vi "atm1.vi"() -> ()   [LabVIEW 2021]
uses:
  Control 8.ctl
  <vilib>/Utility/miscctls.llb/LVPointTypeDef.ctl
panel:
  in  "停止":bool
  in  "插入卡片":bool caption="Card"
  in  "密碼":string
  in  "error in (no error)":errorcluster
  out "error out":errorcluster
  in  "取消":bool
  in  "登入":bool
  in  "帳戶":bool
  in  "領取":bool
  in  "存入":bool
  in  "Money":i32
  out "提示和信息":string
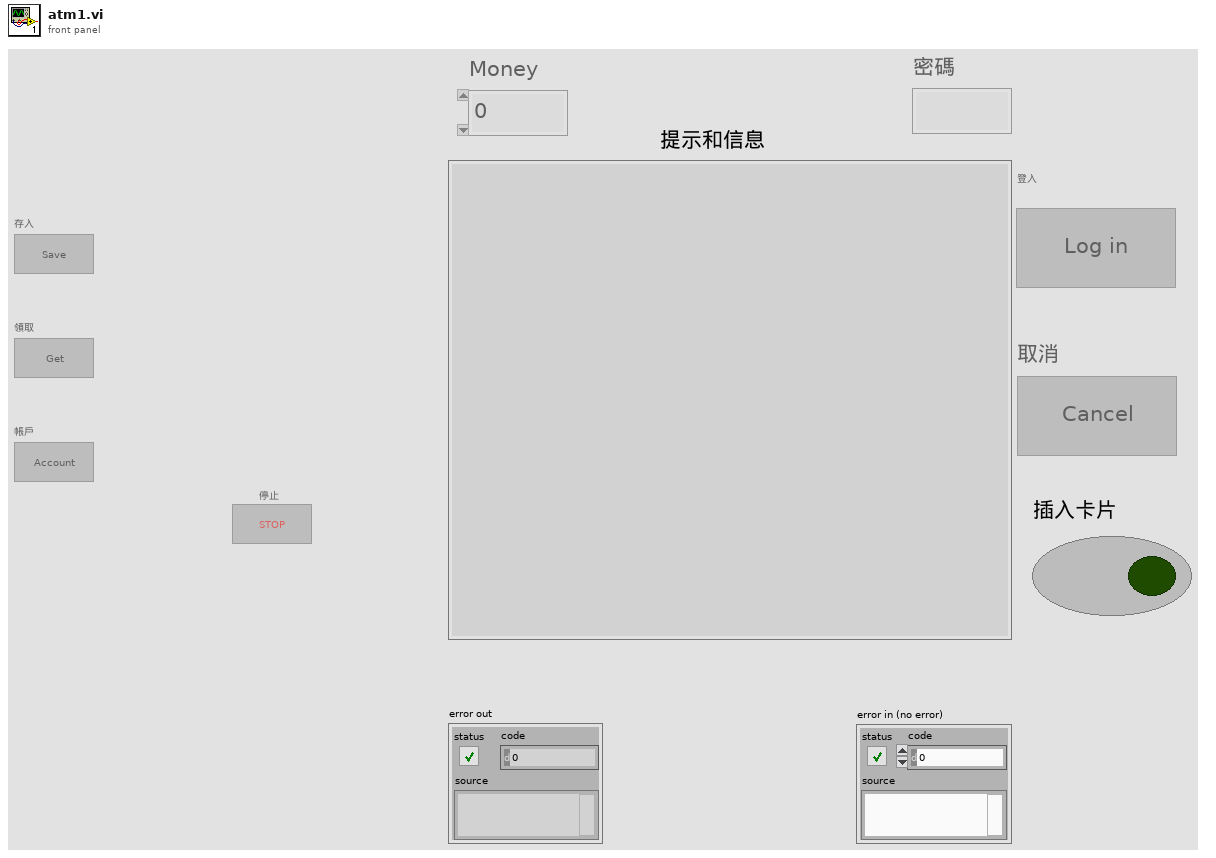
[diagram p1: front panel]
types:
  T1 = typedef "Control 8.ctl" = enum16{"初始化", "調整按鈕狀態", "等待事件", "插入卡片", "登入成功", "密碼錯誤", "密碼連續錯誤", "提款檢查", "提款成功", "提款失敗", "存款", "查詢帳戶餘額", "取消交易", "更新訊息", "停止程式"}
  T2 = typedef "LVPointTypeDef.ctl" = cluster{"Horizontal":i16, "Vertical":i16}
  T3 = enum16{"Enabled", "Disabled", "Disabled and Grayed Out"}
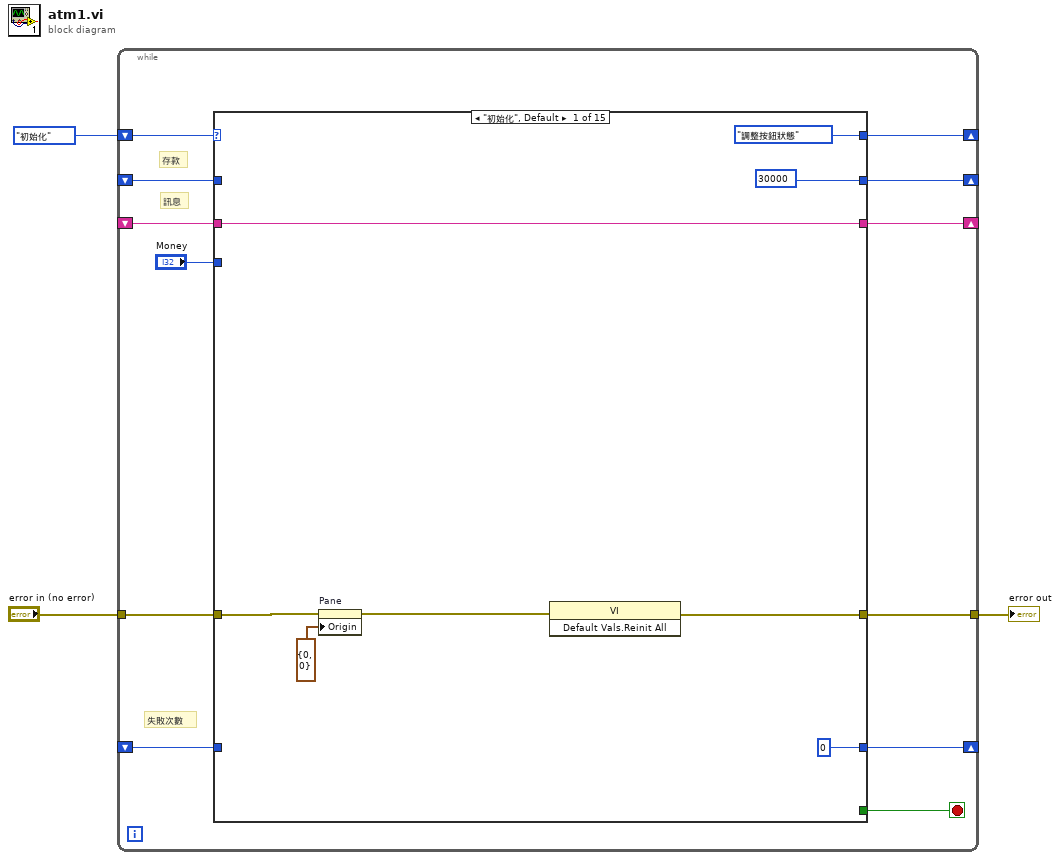
[diagram p0: block diagram]
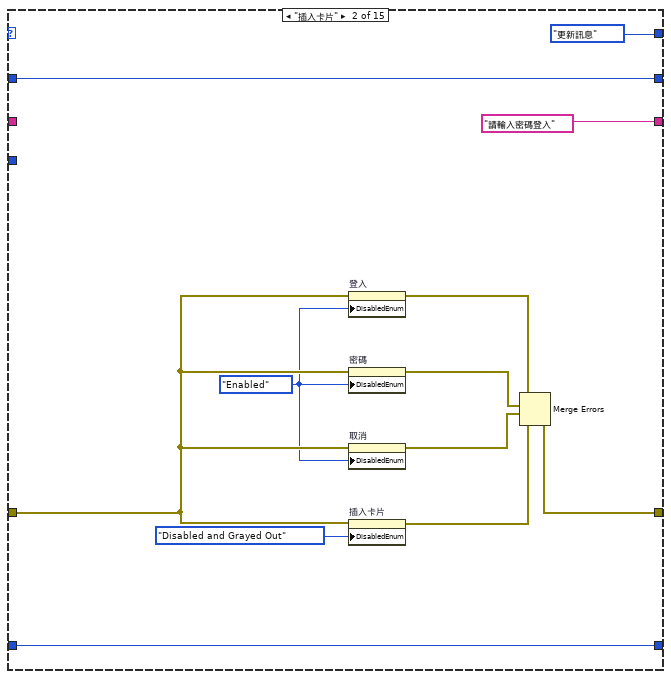
[diagram p2: hidden frame]
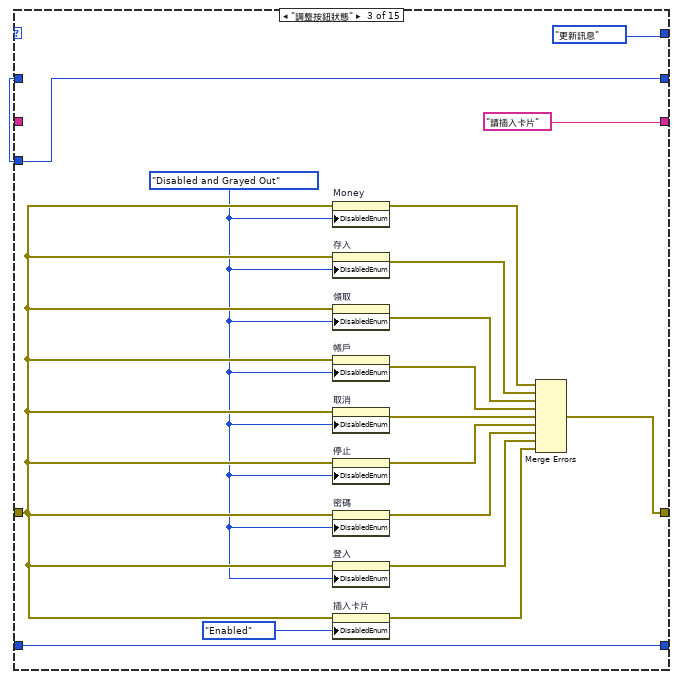
[diagram p3: hidden frame]
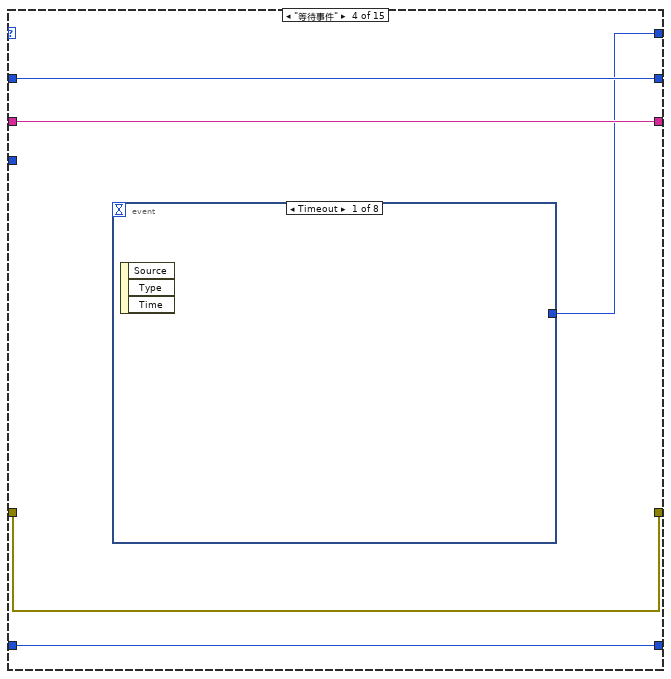
[diagram p4: hidden frame]
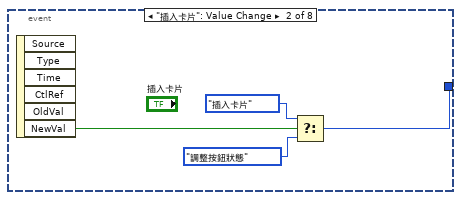
[diagram p5: hidden frame]
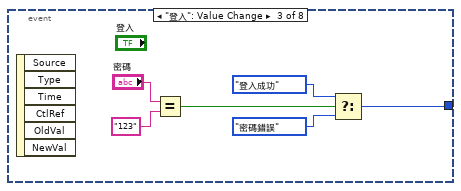
[diagram p6: hidden frame]
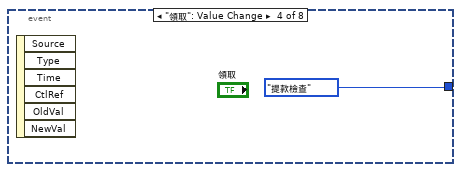
[diagram p7: hidden frame]
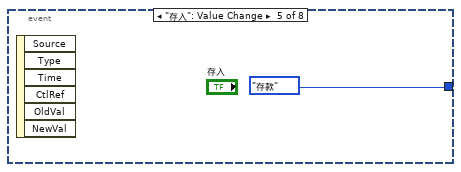
[diagram p8: hidden frame]
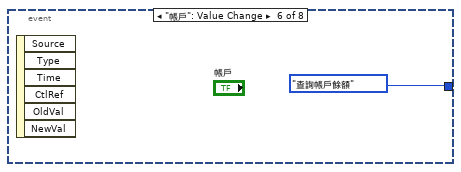
[diagram p9: hidden frame]
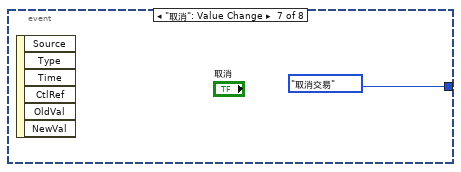
[diagram p10: hidden frame]
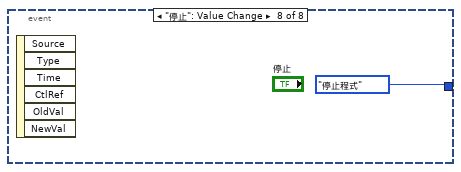
[diagram p11: hidden frame]
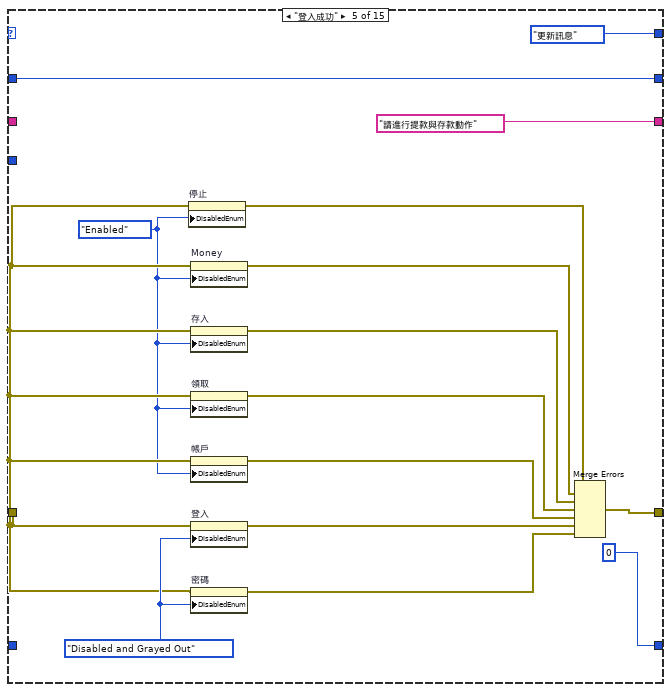
[diagram p12: hidden frame]
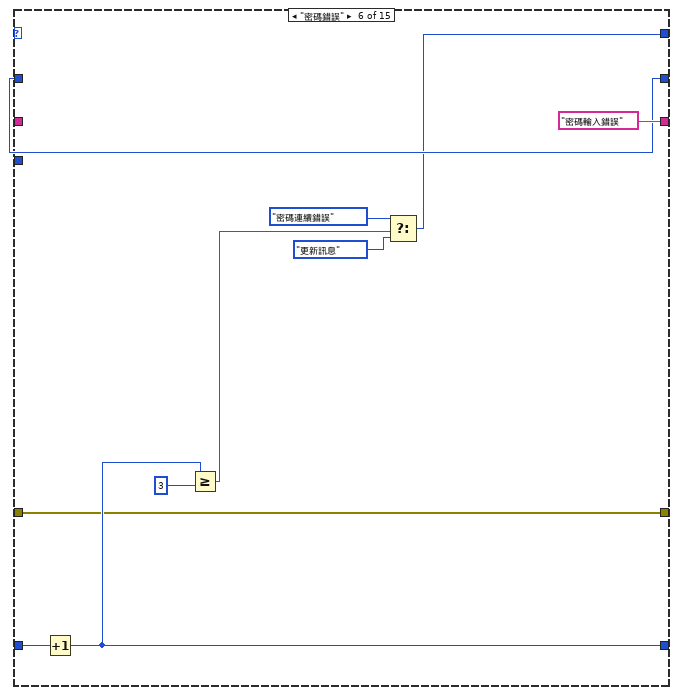
[diagram p13: hidden frame]
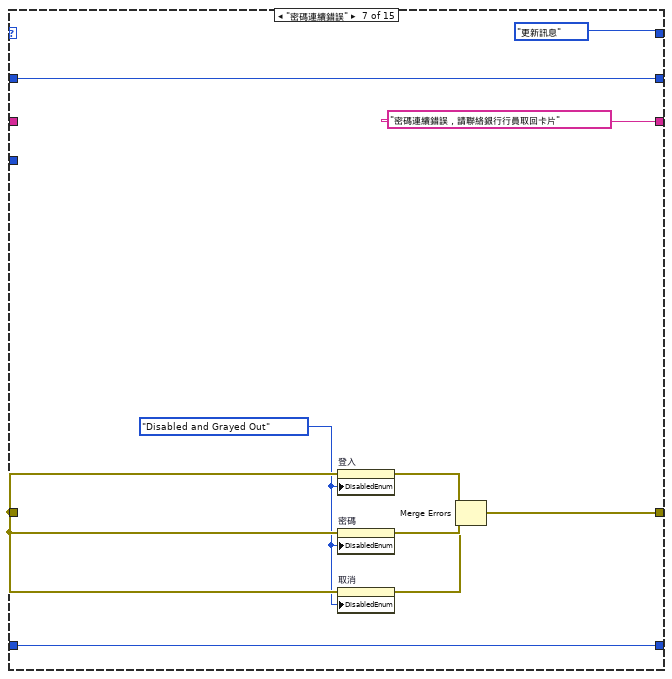
[diagram p14: hidden frame]
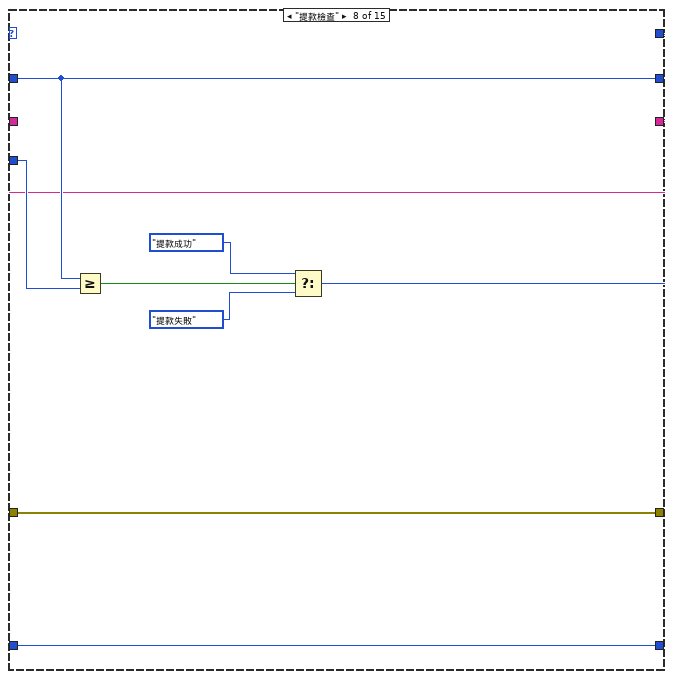
[diagram p15: hidden frame]
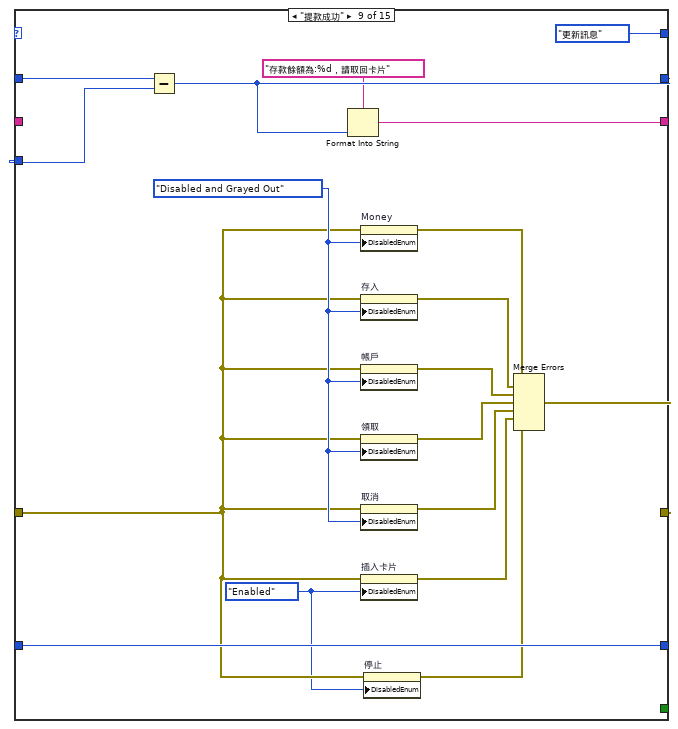
[diagram p16: hidden frame]
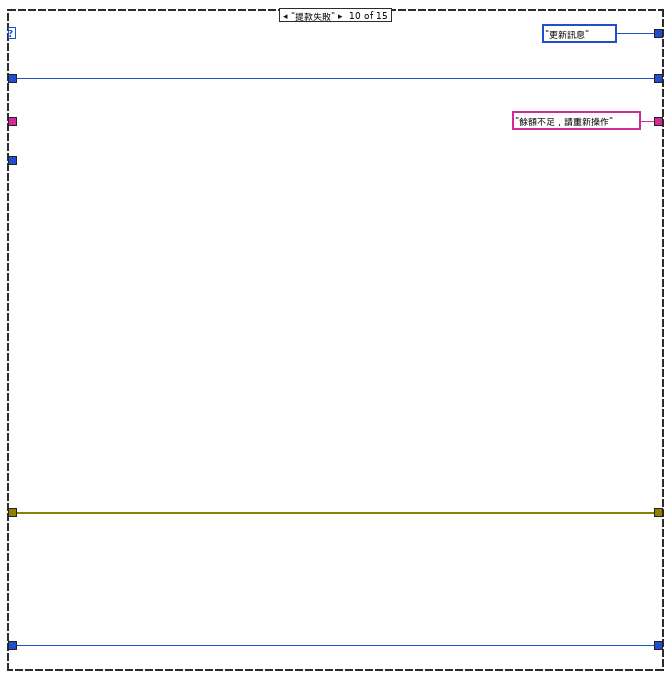
[diagram p17: hidden frame]
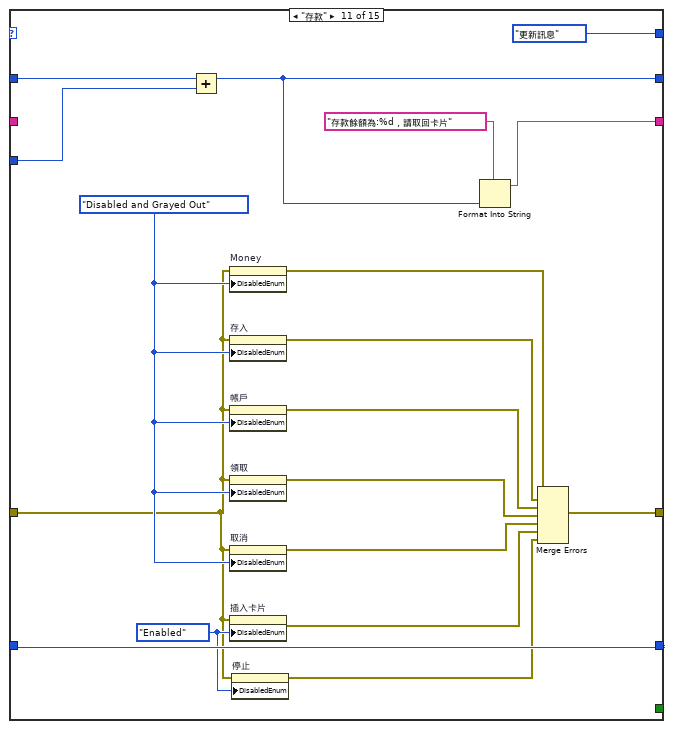
[diagram p18: hidden frame]
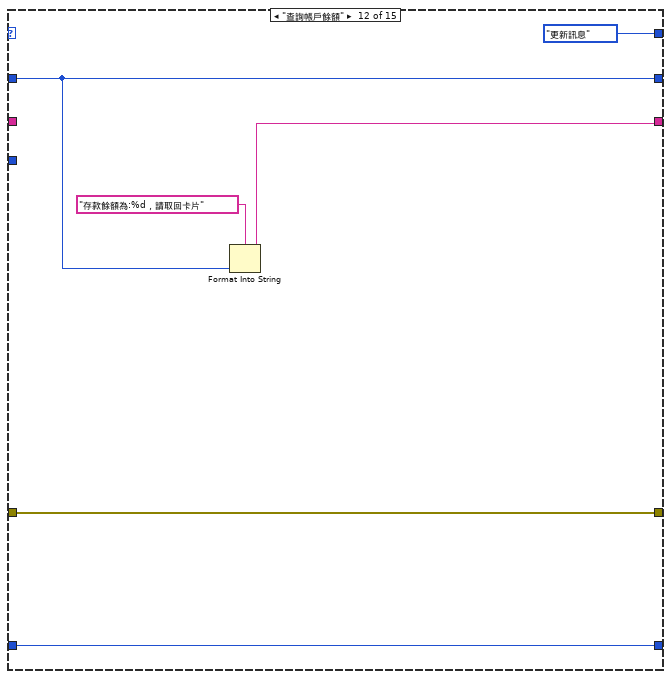
[diagram p19: hidden frame]
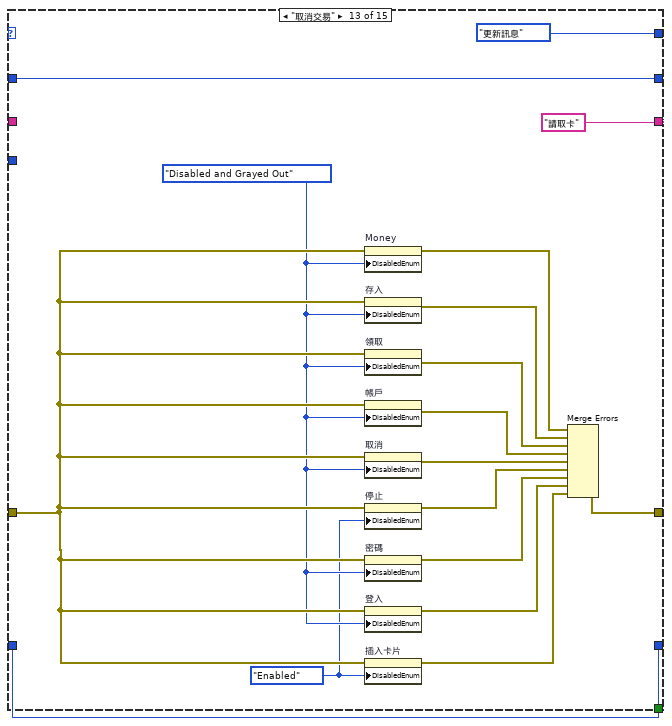
[diagram p20: hidden frame]
diagram:
  n1 = while {
    tunnel: "error in (no error)" -> [w9]
    shift-right: [w12] -> _
    shift-left: _ -> [w15]
    shift-right: [w8] -> _
    shift-left: _ -> [w14]
    shift-right: [w13] -> _
    shift-left: _ -> [w7]
    tunnel: [w10] -> w2
    shift-right: [w5] -> _
    shift-left: Control_8."初始化" -> [w6]
    stop <- w4 stop-if-true
    # "存款"
    # "訊息"
    # "失敗次數"
    n2 = case shown="\"初始化\", Default" w6 {
      selector: w6 -> [_ _ _ _ _ _ _ _ _ _ _ _ _ _ w194]
      tunnel: w15 -> [_ w30 w38 w55 w87 w92 w107 w113 w127 w138 w156 w160 w168 w187 w193]
      tunnel: w14 -> [w17 _ _ w54 _ _ _ w110 _ _ _ _ _ w185 w192]
      tunnel: [0 w27 w40 w57 0 w94 w99 w108 w129 w135 w144 w158 w169 w183 w189] -> w13
      tunnel: [30000 w30 w38 w55 w87 w92 w107 w113 w125 w138 w152 w160 w168 w187 w193] -> w12
      tunnel: "Money" -> [_ _ _ _ _ _ _ w114 w126 _ w155 _ _ _ _]
      tunnel: [w22 w26 w41 w56 w77 w90 w102 w109 w128 w136 w145 w159 w170 w184 w190] -> w10
      tunnel: w9 -> [w21 w35 w51 w56 w74 w90 w106 w109 w120 w136 w141 w159 w171 w184 w191]
      tunnel: [w17 "請輸入密碼登入" "請插入卡片" w54 "請進行提款與存款動作" "密碼輸入錯誤" "密碼連續錯誤，請聯絡銀行行員取回卡片" w110 w123 "餘額不足，請重新操作" w154 w161 "請取卡" w185 w192] -> w8
      tunnel: w7 -> [_ w27 w40 w57 _ w95 w99 w108 w129 w135 w144 w158 w169 w183 w189]
      tunnel: [Control_8."調整按鈕狀態" Control_8."更新訊息" Control_8."更新訊息" w53 Control_8."更新訊息" w91 Control_8."更新訊息" w111 Control_8."更新訊息" Control_8."更新訊息" Control_8."更新訊息" Control_8."更新訊息" Control_8."更新訊息" Control_8."等待事件" w194] -> w5
      tunnel: [_ _ _ _ _ _ _ _ _ _ _ _ _ _ TRUE] -> w4
      frame "初始化", Default {
        n3 = property on="Pane" class="Pane"(error in=w21, "Origin"=T2 {"Horizontal"=0, "Vertical"=0}) -> (error out=w20:errorcluster)  [unwired: 1 in, 1 out]
        n4 = invoke class="VI" method="Default Vals.Reinit All"(error in=w20) -> (error out=w22:errorcluster)  [unwired: 2 in, 2 out]
      }
      frame "插入卡片" {
        w25 = T3."Enabled"
        n5 = property on="登入" class="Bool"(error in=w35, "DisabledEnum"=w25) -> (error out=w34:errorcluster)  [unwired: 1 in, 1 out]
        n6 = property on="密碼" class="Str"(error in=w35, "DisabledEnum"=w25) -> (error out=w33:errorcluster)  [unwired: 1 in, 1 out]
        n7 = property on="取消" class="Bool"(error in=w35, "DisabledEnum"=w25) -> (error out=w32:errorcluster)  [unwired: 1 in, 1 out]
        n8 = property on="插入卡片" class="Bool (strict)"(error in=w35, "DisabledEnum"=T3."Disabled and Grayed Out") -> (error out=w31:errorcluster)  [unwired: 1 in, 1 out]
        n9 = Merge Errors(w34, w33, w32, w31) -> (w26:errorcluster)
      }
      frame "調整按鈕狀態" {
        w36 = T3."Disabled and Grayed Out"
        n10 = property on="Money" class="DigNum (strict)"(error in=w51, "DisabledEnum"=w36) -> (error out=w50:errorcluster)  [unwired: 1 in, 1 out]
        n11 = property on="存入" class="Bool"(error in=w51, "DisabledEnum"=w36) -> (error out=w49:errorcluster)  [unwired: 1 in, 1 out]
        n12 = property on="領取" class="Bool"(error in=w51, "DisabledEnum"=w36) -> (error out=w48:errorcluster)  [unwired: 1 in, 1 out]
        n13 = property on="帳戶" class="Bool"(error in=w51, "DisabledEnum"=w36) -> (error out=w47:errorcluster)  [unwired: 1 in, 1 out]
        n14 = property on="取消" class="Bool"(error in=w51, "DisabledEnum"=w36) -> (error out=w46:errorcluster)  [unwired: 1 in, 1 out]
        n15 = property on="停止" class="Bool"(error in=w51, "DisabledEnum"=w36) -> (error out=w45:errorcluster)  [unwired: 1 in, 1 out]
        n16 = property on="密碼" class="Str"(error in=w51, "DisabledEnum"=w36) -> (error out=w44:errorcluster)  [unwired: 1 in, 1 out]
        n17 = property on="登入" class="Bool"(error in=w51, "DisabledEnum"=w36) -> (error out=w43:errorcluster)  [unwired: 1 in, 1 out]
        n18 = property on="插入卡片" class="Bool (strict)"(error in=w51, "DisabledEnum"=T3."Enabled") -> (error out=w42:errorcluster)  [unwired: 1 in, 1 out]
        n19 = Merge Errors(w50, w49, w48, w47, w46, w45, w44, w43, w42) -> (w41:errorcluster)
      }
      frame "等待事件" {
        n20 = event shown="[0] Timeout" {
          selector: _ -> [_ _ _ _ _ _ _ _]
          dyn-events: _ -> [_ _ _ _ _ _ _ _]
          timeout: _ -> [_ _ _ _ _ _ _ _]
          tunnel: [_ w58 w62 Control_8."提款檢查" Control_8."存款" Control_8."查詢帳戶餘額" Control_8."取消交易" Control_8."停止程式"] -> w53
          event Timeout {
            n21 = event-data() -> ()  [unwired: 1 in, 3 out]
          }
          event "插入卡片": Value Change {
            n22 = event-data() -> ("NewVal"=w59:bool)  [unwired: 1 in, 5 out]
            n23 = Select(t=Control_8."插入卡片", s=w59, f=Control_8."調整按鈕狀態") -> (s? t:f=w58:T1)
          }
          event "登入": Value Change {
            n24 = event-data() -> ()  [unwired: 1 in, 6 out]
            n25 = Equal?(x="密碼", y="123") -> (x = y?=w63:bool)
            n26 = Select(t=Control_8."登入成功", s=w63, f=Control_8."密碼錯誤") -> (s? t:f=w62:T1)
          }
          event "領取": Value Change {
            n27 = event-data() -> ()  [unwired: 1 in, 6 out]
          }
          event "存入": Value Change {
            n28 = event-data() -> ()  [unwired: 1 in, 6 out]
          }
          event "帳戶": Value Change {
            n29 = event-data() -> ()  [unwired: 1 in, 6 out]
          }
          event "取消": Value Change {
            n30 = event-data() -> ()  [unwired: 1 in, 6 out]
          }
          event "停止": Value Change {
            n31 = event-data() -> ()  [unwired: 1 in, 6 out]
          }
        }
      }
      frame "登入成功" {
        w76 = T3."Disabled and Grayed Out"
        w73 = T3."Enabled"
        n32 = property on="停止" class="Bool"(error in=w74, "DisabledEnum"=w73) -> (error out=w75:errorcluster)  [unwired: 1 in, 1 out]
        n33 = property on="Money" class="DigNum (strict)"(error in=w74, "DisabledEnum"=w73) -> (error out=w84:errorcluster)  [unwired: 1 in, 1 out]
        n34 = property on="存入" class="Bool"(error in=w74, "DisabledEnum"=w73) -> (error out=w83:errorcluster)  [unwired: 1 in, 1 out]
        n35 = property on="領取" class="Bool"(error in=w74, "DisabledEnum"=w73) -> (error out=w82:errorcluster)  [unwired: 1 in, 1 out]
        n36 = property on="帳戶" class="Bool"(error in=w74, "DisabledEnum"=w73) -> (error out=w81:errorcluster)  [unwired: 1 in, 1 out]
        n37 = property on="登入" class="Bool"(error in=w74, "DisabledEnum"=w76) -> (error out=w80:errorcluster)  [unwired: 1 in, 1 out]
        n38 = property on="密碼" class="Str"(error in=w74, "DisabledEnum"=w76) -> (error out=w79:errorcluster)  [unwired: 1 in, 1 out]
        n39 = Merge Errors(w75, w84, w83, w82, w81, w80, w79) -> (w77:errorcluster)
      }
      frame "密碼錯誤" {
        n40 = Increment(x=w95) -> (x+1=w94:i32)
        n41 = Greater Or Equal?(x=w94, y=3) -> (x >= y?=w93:bool)
        n42 = Select(t=Control_8."密碼連續錯誤", s=w93, f=Control_8."更新訊息") -> (s? t:f=w91:T1)
      }
      frame "密碼連續錯誤" {
        w98 = T3."Disabled and Grayed Out"
        n43 = property on="登入" class="Bool"(error in=w106, "DisabledEnum"=w98) -> (error out=w105:errorcluster)  [unwired: 1 in, 1 out]
        n44 = property on="密碼" class="Str"(error in=w106, "DisabledEnum"=w98) -> (error out=w104:errorcluster)  [unwired: 1 in, 1 out]
        n45 = property on="取消" class="Bool"(error in=w106, "DisabledEnum"=w98) -> (error out=w103:errorcluster)  [unwired: 1 in, 1 out]
        n46 = Merge Errors(w105, w104, w103) -> (w102:errorcluster)
      }
      frame "提款檢查" {
        n47 = Greater Or Equal?(x=w113, y=w114) -> (x >= y?=w112:bool)
        n48 = Select(t=Control_8."提款成功", s=w112, f=Control_8."提款失敗") -> (s? t:f=w111:T1)
      }
      frame "提款成功" {
        w121 = T3."Disabled and Grayed Out"
        w119 = T3."Enabled"
        n49 = Subtract(x=w127, y=w126) -> (x-y=w125:i32)
        n50 = Format Into String(format string="存款餘額為:%d，請取回卡片", w125) -> (resulting string=w123:string)  [unwired: 2 in, 1 out]
        n51 = property on="Money" class="DigNum (strict)"(error in=w120, "DisabledEnum"=w121) -> (error out=w134:errorcluster)  [unwired: 1 in, 1 out]
        n52 = property on="存入" class="Bool"(error in=w120, "DisabledEnum"=w121) -> (error out=w133:errorcluster)  [unwired: 1 in, 1 out]
        n53 = property on="帳戶" class="Bool"(error in=w120, "DisabledEnum"=w121) -> (error out=w132:errorcluster)  [unwired: 1 in, 1 out]
        n54 = property on="領取" class="Bool"(error in=w120, "DisabledEnum"=w121) -> (error out=w131:errorcluster)  [unwired: 1 in, 1 out]
        n55 = property on="取消" class="Bool"(error in=w120, "DisabledEnum"=w121) -> (error out=w130:errorcluster)  [unwired: 1 in, 1 out]
        n56 = property on="插入卡片" class="Bool (strict)"(error in=w120, "DisabledEnum"=w119) -> (error out=w118:errorcluster)  [unwired: 1 in, 1 out]
        n57 = property on="停止" class="Bool"(error in=w120, "DisabledEnum"=w119) -> (error out=w117:errorcluster)  [unwired: 1 in, 1 out]
        n58 = Merge Errors(w134, w133, w132, w131, w130, w118, w117) -> (w128:errorcluster)
      }
      frame "提款失敗" {
      }
      frame "存款" {
        w142 = T3."Enabled"
        w143 = T3."Disabled and Grayed Out"
        n59 = Add(x=w156, y=w155) -> (x+y=w152:i32)
        n60 = property on="Money" class="DigNum (strict)"(error in=w141, "DisabledEnum"=w143) -> (error out=w151:errorcluster)  [unwired: 1 in, 1 out]
        n61 = property on="存入" class="Bool"(error in=w141, "DisabledEnum"=w143) -> (error out=w150:errorcluster)  [unwired: 1 in, 1 out]
        n62 = property on="帳戶" class="Bool"(error in=w141, "DisabledEnum"=w143) -> (error out=w149:errorcluster)  [unwired: 1 in, 1 out]
        n63 = property on="領取" class="Bool"(error in=w141, "DisabledEnum"=w143) -> (error out=w148:errorcluster)  [unwired: 1 in, 1 out]
        n64 = property on="取消" class="Bool"(error in=w141, "DisabledEnum"=w143) -> (error out=w147:errorcluster)  [unwired: 1 in, 1 out]
        n65 = property on="插入卡片" class="Bool (strict)"(error in=w141, "DisabledEnum"=w142) -> (error out=w146:errorcluster)  [unwired: 1 in, 1 out]
        n66 = property on="停止" class="Bool"(error in=w141, "DisabledEnum"=w142) -> (error out=w140:errorcluster)  [unwired: 1 in, 1 out]
        n67 = Format Into String(format string="存款餘額為:%d，請取回卡片", w152) -> (resulting string=w154:string)  [unwired: 2 in, 1 out]
        n68 = Merge Errors(w151, w150, w149, w148, w147, w146, w140) -> (w145:errorcluster)
      }
      frame "查詢帳戶餘額" {
        n69 = Format Into String(format string="存款餘額為:%d，請取回卡片", w160) -> (resulting string=w161:string)  [unwired: 2 in, 1 out]
      }
      frame "取消交易" {
        w165 = T3."Disabled and Grayed Out"
        w164 = T3."Enabled"
        n70 = property on="Money" class="DigNum (strict)"(error in=w171, "DisabledEnum"=w165) -> (error out=w180:errorcluster)  [unwired: 1 in, 1 out]
        n71 = property on="存入" class="Bool"(error in=w171, "DisabledEnum"=w165) -> (error out=w179:errorcluster)  [unwired: 1 in, 1 out]
        n72 = property on="領取" class="Bool"(error in=w171, "DisabledEnum"=w165) -> (error out=w178:errorcluster)  [unwired: 1 in, 1 out]
        n73 = property on="帳戶" class="Bool"(error in=w171, "DisabledEnum"=w165) -> (error out=w177:errorcluster)  [unwired: 1 in, 1 out]
        n74 = property on="取消" class="Bool"(error in=w171, "DisabledEnum"=w165) -> (error out=w176:errorcluster)  [unwired: 1 in, 1 out]
        n75 = property on="停止" class="Bool"(error in=w171, "DisabledEnum"=w164) -> (error out=w175:errorcluster)  [unwired: 1 in, 1 out]
        n76 = property on="密碼" class="Str"(error in=w171, "DisabledEnum"=w165) -> (error out=w174:errorcluster)  [unwired: 1 in, 1 out]
        n77 = property on="登入" class="Bool"(error in=w171, "DisabledEnum"=w165) -> (error out=w173:errorcluster)  [unwired: 1 in, 1 out]
        n78 = property on="插入卡片" class="Bool (strict)"(error in=w171, "DisabledEnum"=w164) -> (error out=w172:errorcluster)  [unwired: 1 in, 1 out]
        n79 = Merge Errors(w180, w179, w178, w177, w176, w175, w174, w173, w172) -> (w170:errorcluster)
      }
      frame "更新訊息" {
        n80 = local write "Money"(0) -> ()
        n81 = local write "密碼"("") -> ()
        "提示和信息" <- w185
      }
      frame "停止程式" {
        n82 = invoke class="VI" method="Default Vals.Reinit All"(error in=w191) -> (error out=w190:errorcluster)  [unwired: 2 in, 2 out]
      }
    }
  }
  "error out" <- w2
